vi "setBounds.vi"(0 "reference":refnum<class "RectangularNode.lvclass">, 1 "bounds":T1 {"height" format="%.2f"; "width" format="%.2f"; "y" format="%.2f"; "x" format="%.2f"}, 5 "error in (no error)":errorcluster) -> (14 "reference out":refnum<class "RectangularNode.lvclass">, 19 "error out":errorcluster)   [LabVIEW 2014, in "RectangularNode.lvclass"]
doc: "public void setBounds(Rectangle2D newBounds)"
uses:
  <resource>/Framework/Providers/Open_GDS/UML/RectangularNode_class/RectangularNode.lvclass
  <resource>/Framework/Providers/Open_GDS/UML/General/Rectangle/Rectangle Rectangle2D.ctl
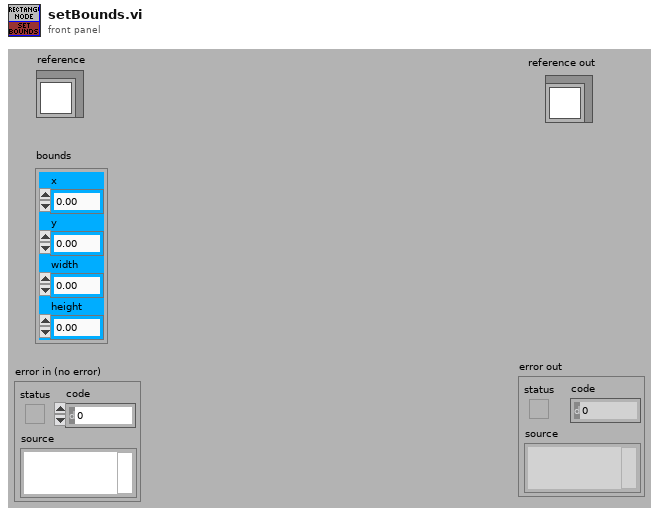
[diagram p1: front panel]
types:
  T1 = typedef "Rectangle Rectangle2D.ctl" = cluster{"x":dbl, "y":dbl, "width":dbl, "height":dbl}
  T2 = typedef "RectangularNode.lvclass/ObjectAttributes.ctl" = cluster{"Base class":T3, "bounds":T1}
  T3 = typedef "AbstractNode.lvclass/ObjectAttributes.ctl" = cluster{"parent":refnum<class "AbstractNode.lvclass">, "children":refnum<class "AbstractNode.lvclass">[], "Hidden":bool}
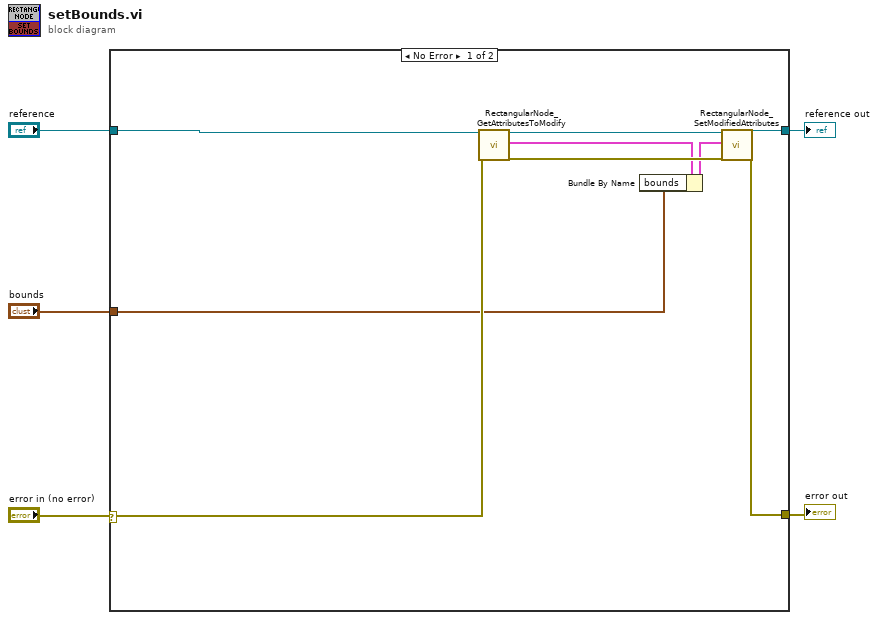
[diagram p0: block diagram]
diagram:
  n1 = case shown="No Error" "error in (no error)" {
    selector: "error in (no error)" -> [w11 w15]
    tunnel: "reference" -> [w14 w16]
    tunnel: [w13 w15] -> w4
    tunnel: [w12 w16] -> w3
    tunnel: "bounds" -> [w10 _]
    frame No Error {
      n2 = call <resource>:"RectangularNode_GetAttributesToModify.vi"("reference in"=w14, "error in (no error)"=w11) -> ("reference out"=w8:refnum<class "RectangularNode.lvclass">, "Attributes"=w7:T2, "error out"=w9:errorcluster)  [unwired: 1 in, 14 out]
      n3 = Bundle By Name(cluster=w7, "bounds"=w10) -> (w6:T2)
      n4 = call <resource>:"RectangularNode_SetModifiedAttributes.vi"("reference in"=w8, "Attributes"=w6, "error in (no error)"=w9) -> ("reference out"=w12:refnum<class "RectangularNode.lvclass">, "error out"=w13:errorcluster)  [unwired: 3 in, 12 out]
    }
    frame Error {
    }
  }
  "reference out" <- w3
  "error out" <- w4
